vi "Overload Counter Channels Write Array.vi"(8 "error in":errorcluster, 10 "Overload Counter AV":dbl[](array[numeric]), 11 "Overload Counter Channels in":refnum<class "Overload Counter Channels.lvclass">) -> (0 "error out":errorcluster, 3 "Overload Counter Channels out":refnum<class "Overload Counter Channels.lvclass">)   [LabVIEW 2023, in "Overload Counter Channels.lvclass"]
uses:
  Overload Counter Channels.lvclass
  Overload Counter Channels.lvclass/Overload Counter Channels.ctl
  <vilib>/ADAS Replay HIL/Channels/Tag Wrapper/Polymorphic/Write Channel (Double).vi
  <vilib>/ADAS Replay HIL/Channels/Tag Wrapper/Polymorphic/Write Channel (Double).vi/cccb8e89-591f-4bb4-9d4e-ae06ba1f5498.vi
  <vilib>/ADAS Replay HIL/Channels/Tag Wrapper/Polymorphic/Write Channel (Double).vi/cccb8e89-591f-4bb4-9d4e-ae06ba1f5498.vi/4bc1c15b-36ab-481f-b8dd-c64075ce723a.vi
  <vilib>/ADAS Replay HIL/Channels/Tag Wrapper/Polymorphic/Write Channel (Double).vi/cccb8e89-591f-4bb4-9d4e-ae06ba1f5498.vi/d83cb72b-7713-41fc-a3d1-682de79cf574.vi
  <vilib>/ADAS Replay HIL/Channels/Tag Wrapper/Tag Wrapper.lvlib
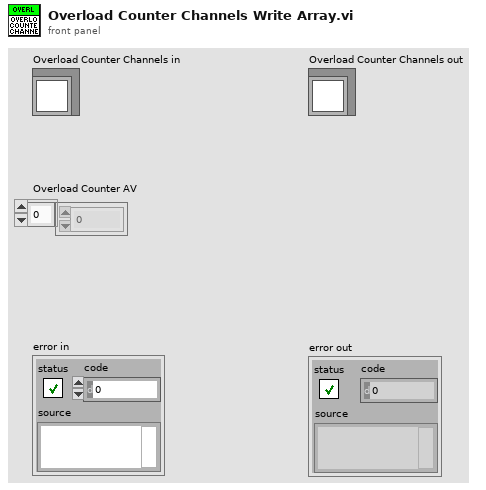
[diagram p1: front panel]
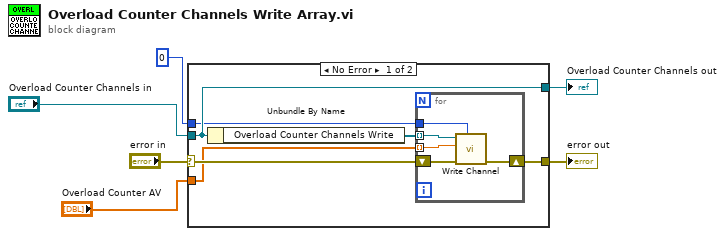
[diagram p0: block diagram]
diagram:
  n1 = case shown="No Error" "error in" {
    selector: "error in" -> [w12 w19]
    tunnel: [w11 w19] -> w5
    tunnel: [w9 w18] -> w1
    tunnel: "Overload Counter Channels in" -> [w9 w18]
    tunnel: "Overload Counter AV" -> [w8 _]
    tunnel: 0 ("Timeout (ms)") -> [w7 _]
    frame No Error {
      n2 = Unbundle By Name(w9) -> ("Overload Counter Channels Write"=w10:refnum<k21>[])
      n3 = for {
        shift-right: [w16] -> w11
        shift-left: w12 -> [w17]
        tunnel: w10 -> [w15] mode=indexing
        tunnel: w8 -> [w14] mode=indexing
        tunnel: w7 -> [w13]
        n4 = call-poly <vilib>:"Write Channel.vi"("Timeout (ms)"=w13, "error in"=w17, "Value to Write"=w14, "ADAS HIL Channel in"=w15) -> ("error out"=w16:errorcluster)  [unwired: 5 in, 2 out]
      }
    }
    frame Error {
    }
  }
  "error out" <- w5
  "Overload Counter Channels out" <- w1
